vi "Stop.vi"(8 "error in (no error)":errorcluster, 10 "switch lamp off (true)":bool=TRUE, 11 "Lotis in":refnum<class "PL Lotis TII LS.lvclass">) -> (0 "error out":errorcluster, 3 "Lotis out":refnum<class "PL Lotis TII LS.lvclass">)   [LabVIEW 2015, in "PL Lotis TII LS.lvclass"]
doc: "Stops generation."
uses:
  PL Lotis TII LS.lvclass
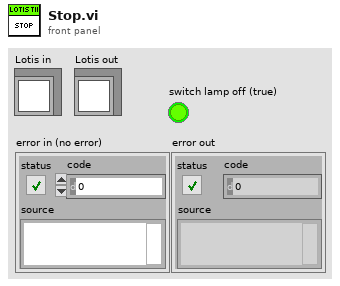
[diagram p1: front panel]
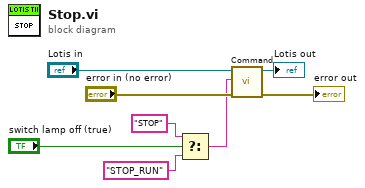
[diagram p0: block diagram]
diagram:
  n1 = Select(t="STOP" ("command"), s="switch lamp off (true)", f="STOP_RUN" ("command")) -> (s? t:f=w1:string)
  n2 = call "Command.vi"("error in (no error)"="error in (no error)", "command"=w1, "Lotis in"="Lotis in") -> ("error out"=→"error out":errorcluster, "Lotis out"=→"Lotis out":refnum<class "PL Lotis TII LS.lvclass">)  [unwired: 6 in, 1 out]
